vi "Configure Trigger Delay.vi"(7 "Delay Time (0 s)":dbl, 8 "error in (no error)":errorcluster, 9 "Channel Mode (0: Single)":i32(ring) items=["Single", "Dual"], 10 "Analyzer (0: A0)":i32(ring) items=["A0", "A1"], 11 "VISA resource name":refnum<visa-resource-name>) -> (0 "error out":errorcluster, 3 "VISA resource name out":refnum<visa-resource-name>)   [LabVIEW 2014, in "Stanford Research SR1.lvlib"]
doc: "Configures the attributes for the Trigger Delay."
uses:
  Stanford Research SR1.lvlib
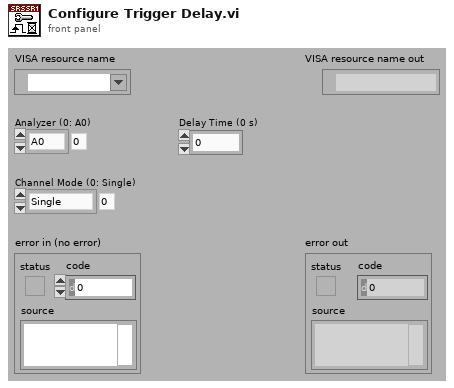
[diagram p1: front panel]
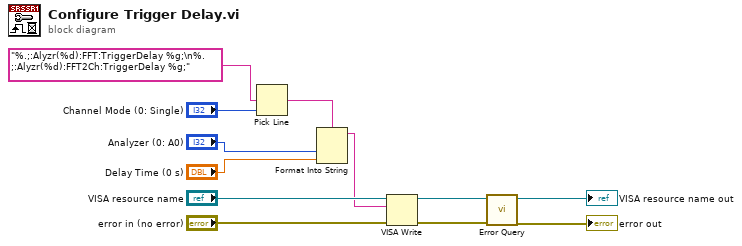
[diagram p0: block diagram]
diagram:
  n1 = Pick Line(multi-line string="%.;:Alyzr(%d):FFT:TriggerDelay %g;\n%.;:Alyzr(%d):FFT2Ch:TriggerDelay %g;", line index="Channel Mode (0: Single)") -> (output string=w4:string)  [unwired: 1 in]
  n2 = Format Into String(format string=w4, "Analyzer (0: A0)", "Delay Time (0 s)") -> (resulting string=w1:string)  [unwired: 2 in, 1 out]
  n3 = VISA Write(VISA resource name="VISA resource name", write buffer=w1, error in (no error)="error in (no error)") -> (VISA resource name out=w10:refnum<visa-resource-name>, error out=w9:errorcluster)  [unwired: 1 out]
  n4 = call "Error Query.vi"("error in (no error)"=w9, "VISA resource name"=w10) -> ("error out"=→"error out":errorcluster, "VISA resource name out"=→"VISA resource name out":refnum<visa-resource-name>)  [unwired: 6 in, 2 out]
